vi "SetParam.vi"(6 "DAQmx Device Name":tag, 7 "RS":bool, 8 "error in (no error)":errorcluster, 9 "Param to Set in":u16, 10 "Visa":refnum<visa-resource-name>, 11 "Filein":string) -> (0 "error out":errorcluster)   [LabVIEW 2017]
uses:
  <vilib>/Utility/miscctls.llb/LVMinMaxIncTypeDef.ctl
  <vilib>/Utility/config.llb/NI_LVConfig.lvlib
  <vilib>/Utility/config.llb/Read Key (String).vi
panel:
  out "match substring":string
  out "RS Out":string
  out "Horizontal Progress Bar":i32(slide) min=0 max=32 scale=0.0..50.0
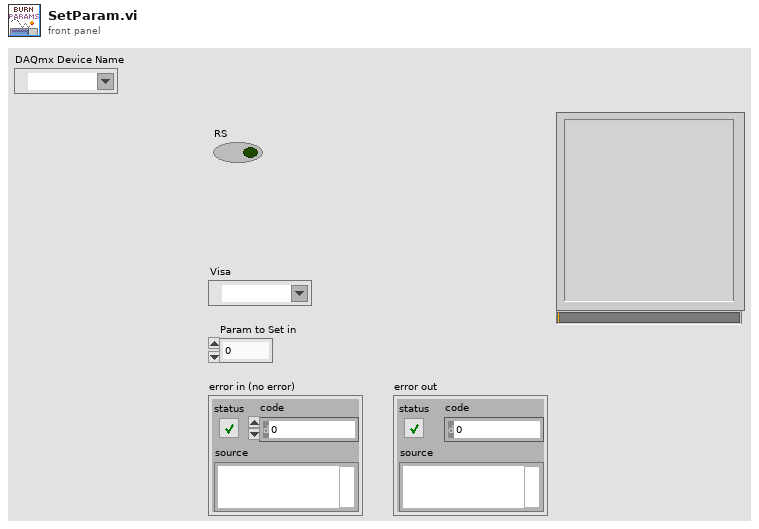
[diagram p1: front panel]
types:
  T1 = typedef "NI_LVConfig.lvlib/Config Data RefNum.ctl" = refnum<k1>
  T2 = typedef "LVMinMaxIncTypeDef.ctl" = cluster{"Minimum":dbl, "Maximum":dbl, "Increment":dbl}
  T3 = cluster{"Action":string, "ON(T)OFF(F)":bool, "Func":enum16{"Init", "VEnable", "PowerOnOff", "PowerONVEnable"}}
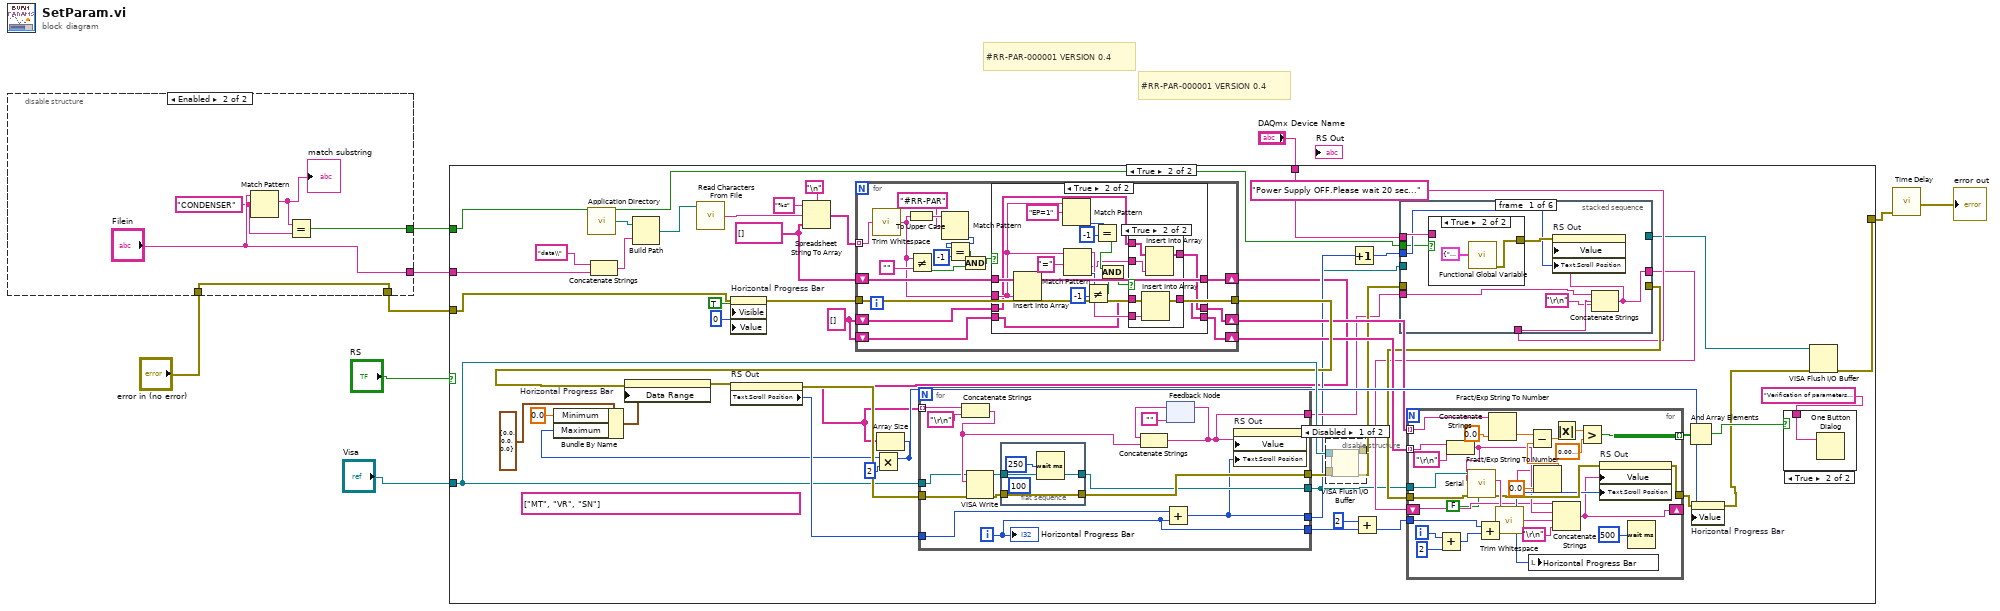
[diagram p0: block diagram]
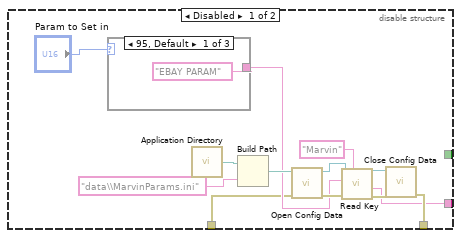
[diagram p2: hidden frame]
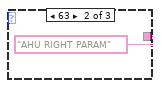
[diagram p3: hidden frame]
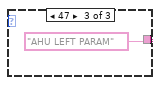
[diagram p4: hidden frame]
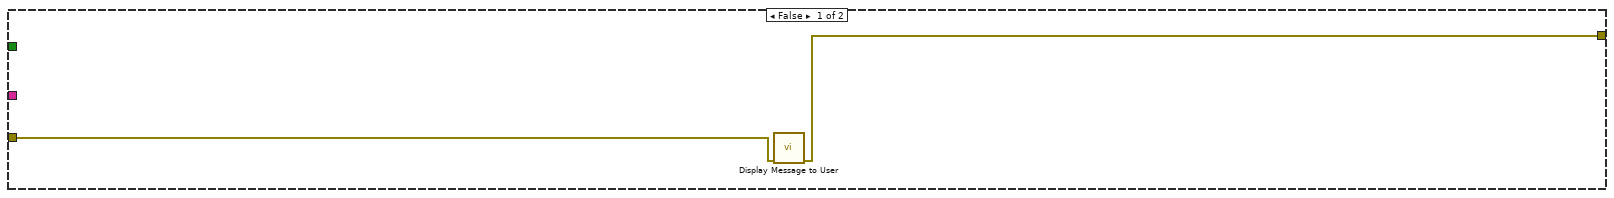
[diagram p5: hidden frame]
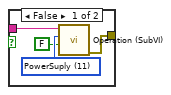
[diagram p7: hidden frame]
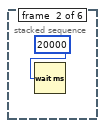
[diagram p8: hidden frame]
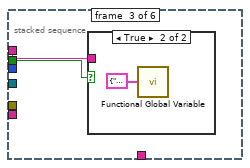
[diagram p9: hidden frame]
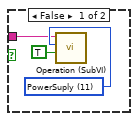
[diagram p10: hidden frame]
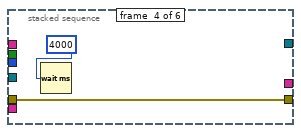
[diagram p11: hidden frame]
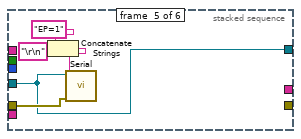
[diagram p12: hidden frame]
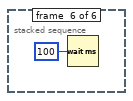
[diagram p13: hidden frame]
diagram:
  # "#RR-PAR-000001 VERSION 0.4"
  # "#RR-PAR-000001 VERSION 0.4"
  n1 = disable-structure shown="Enabled" {
    disable-tunnel: "error in (no error)" -> [w13 w30]
    disable-tunnel: [w12 w30] -> w6
    disable-tunnel: [w11 "Filein"] -> w5
    disable-tunnel: [_ w26] -> w1
    frame Disabled {
      n2 = case shown="95, Default" "Param to Set in" {
        tunnel: ["EBAY PARAM" ("section") "AHU RIGHT PARAM" ("section") "AHU LEFT PARAM" ("section")] -> w14
        frame 95, Default {
        }
        frame 63 {
        }
        frame 47 {
        }
      }
      n3 = call <vilib>:"Application Directory.vi"() -> ("Application Directory"=w22:path)
      n4 = Build Path(base path=w22, name or relative path="data\\MarvinParams.ini") -> (appended path=w18:path)
      n5 = call <vilib>:"Open Config Data.vi"("error in (no error)"=w13, "configuration file path"=w18) -> ("error out"=w17:errorcluster, "refnum"=w20:T1)  [unwired: 1 in, 7 out]
      n6 = call-poly <vilib>:"Read Key.vi"("section"="Marvin", "error in (no error)"=w17, "key"=w14, "refnum"=w20) -> ("error out"=w16:errorcluster, "value"=w11:string, "refnum out"=w15:T1)  [unwired: 2 in, 3 out]
      n7 = call <vilib>:"Close Config Data.vi"("error in (no error)"=w16, "refnum"=w15) -> ("error out"=w12:errorcluster)  [unwired: 8 in, 1 out]
    }
    frame Enabled {
      w27 = "CONDENSER" ("regular expression")
      n8 = Match Pattern(string="Filein", regular expression=w27) -> (match substring=w28:string)  [unwired: 1 in, 3 out]
      "match substring" <- w28
      n9 = Equal?(x=w28, y=w27) -> (x = y?=w26:bool)
    }
  }
  n10 = case shown="True" "RS" {
    tunnel: w6 -> [w32 w72]
    tunnel: [w31 w35] -> w9
    tunnel: "Visa" -> [_ w73]
    tunnel: w5 -> [_ w39]
    tunnel: "DAQmx Device Name" -> [_ w53]
    tunnel: w1 -> [_ w33]
    frame False {
      n11 = call "Display Message to User"("error in (no error)"=w32) -> ("error out"=w31:errorcluster)  [unwired: 9 in, 1 out]
    }
    frame True {
      w59 = string[] []
      w60 = string[] []
      (unwired) string[] ["MT", "VR", "SN"] ("array")
      n12 = call <vilib>:"Application Directory.vi"() -> ("Application Directory"=w70:path)
      n13 = Concatenate Strings("data\\" ("name or relative path"), w39) -> (w71:string)
      n14 = Build Path(base path=w70, name or relative path=w71) -> (appended path=w68:path)
      n15 = call <vilib>:"Read Characters From File.vi"("file path (dialog if empty)"=w68) -> ("character string"=w66:string)  [unwired: 5 in, 3 out]
      n16 = property on="Horizontal Progress Bar" class="Slide (strict)"(error in=w72, "Visible"=TRUE, "Value"=u8 0 ("Horizontal Progress Bar")) -> (error out=w64:errorcluster)  [unwired: 1 in, 1 out]
      n17 = Spreadsheet String To Array(delimiter (Tab)="\n", format string="%s", spreadsheet string=w66, array type (2D Dbl)=w60) -> (array=w65:string[])
      n18 = for {
        tunnel: w65 -> [w159] mode=indexing
        tunnel: w64 -> [w160]
        tunnel: [w160] -> w63
        shift-right: [w157] -> w37
        shift-left: w60 -> [w158]
        shift-right: [w146] -> w58
        shift-left: w59 -> [w147]
        shift-right: [w144] -> w57
        shift-left: w59 -> [w145]
        n19 = call <vilib>:"Trim Whitespace.vi"("string"=w159) -> ("trimmed string"=w148:string)  [unwired: 1 in]
        n20 = To Upper Case(1:w148) -> (0:w156:string)
        n21 = Not Equal?(x=w148, y="") -> (x != y?=w149:bool)
        n22 = Match Pattern(string=w156, regular expression="#RR-PAR") -> (offset past match=w154:i32)  [unwired: 1 in, 3 out]
        n23 = Equal?(x=w154, y=-1) -> (x = y?=w152:bool)
        n24 = And(x=w152, y=w149) -> (x .and. y?=w151:bool)
        n25 = case shown="True" w151 {
          tunnel: w158 -> [w163 w181]
          tunnel: [w163 w180] -> w157
          tunnel: w148 -> [_ w168]
          tunnel: w147 -> [w162 w164]
          tunnel: [w162 w165] -> w146
          tunnel: w145 -> [w161 w167]
          tunnel: [w161 w166] -> w144
          frame False {
          }
          frame True {
            n26 = Insert Into Array(array=w181, new element=w168) -> (w180:string[])  [unwired: 1 in]
            n27 = Match Pattern(string=w168, regular expression="EP=1") -> (offset past match=w177:i32)  [unwired: 1 in, 3 out]
            n28 = Match Pattern(string=w168, regular expression="=") -> (before substring=w178:string, after substring=w173:string, offset past match=w179:i32)  [unwired: 1 in, 1 out]
            n29 = Not Equal?(x=w179, y=-1) -> (x != y?=w176:bool)
            n30 = Equal?(x=w177, y=-1) -> (x = y?=w174:bool)
            n31 = And(x=w174, y=w176) -> (x .and. y?=w175:bool)
            n32 = case shown="True" w175 {
              tunnel: w167 -> [w183 w189]
              tunnel: [w183 w188] -> w166
              tunnel: w178 -> [_ w187]
              tunnel: w173 -> [_ w186]
              tunnel: w164 -> [w182 w185]
              tunnel: [w182 w184] -> w165
              frame False {
              }
              frame True {
                n33 = Insert Into Array(array=w189, new element=w187) -> (w188:string[])  [unwired: 1 in]
                n34 = Insert Into Array(array=w185, new element=w186) -> (w184:string[])  [unwired: 1 in]
              }
            }
          }
        }
      }
      n35 = Array Size(array=w37) -> (size(s)=w67:i32)
      n36 = Multiply(x=w67, y=2) -> (x*y=w50:i32)
      n37 = Bundle By Name(cluster=T2 {"Minimum"=0.0, "Maximum"=0.0, "Increment"=0.0} ("Data Entry Limits"), "Minimum"=0.0, "Maximum"=w50) -> (w79:T2)
      n38 = property on="Horizontal Progress Bar" class="Slide (strict)"(error in=w63, "Data Range"=w79) -> (error out=w76:errorcluster)  [unwired: 1 in, 1 out]
      n39 = property on="RS Out" class="Str"(error in=w76) -> (error out=w75:errorcluster, "Text.Scroll Position"=w74:u32)  [unwired: 1 in, 1 out]
      n40 = for {
        tunnel: w37 -> [w200] mode=indexing
        tunnel: w75 -> [w204]
        tunnel: [w197] -> w77
        tunnel: w74 -> [w196]
        tunnel: w73 -> [w195]
        tunnel: [w193] -> w38
        tunnel: [w192] -> w47
        tunnel: [w191] -> w45
        tunnel: [w190] -> w43
        i -> [w192]
        n41 = Concatenate Strings(w200, "\r\n" ("string")) -> (w198:string)
        n42 = VISA Write(VISA resource name=w195, write buffer=w198, error in (no error)=w204) -> (VISA resource name out=w194:refnum<visa-resource-name>, error out=w203:errorcluster)  [unwired: 1 out]
        n43 = flat-sequence {
          tunnel: w203 -> [w206]
          tunnel: [w206] -> w197
          tunnel: w194 -> [w205]
          tunnel: [w205] -> w193
          frame #0 {
            (unwired) u32 100 ("milliseconds to wait")
            n44 = Wait (ms)(milliseconds to wait=u32 250) -> ()  [unwired: 1 out]
          }
        }
        n45 = Add(x=w196, y=w192) -> (x+y=w190:u32)
        n46 = feedback #1("") -> (w202:string)
        n47 = Concatenate Strings(w202, w198) -> (w191:string)
        n48 = feedback-in #1(w191) -> ()
        n49 = property on="RS Out" class="Str"("Value"=w191, "Text.Scroll Position"=w190) -> ()  [unwired: 2 in, 2 out]
        "Horizontal Progress Bar" <- w192
      }
      n50 = disable-structure shown="Disabled" {
        disable-tunnel: w77 -> [w85 _]
        disable-tunnel: w73 -> [w84 _]
        disable-tunnel: [w83 _] -> w52
        frame Disabled {
          n51 = VISA Flush I/O Buffer(VISA resource name=w84, error in (no error)=w85) -> (error out=w83:errorcluster)  [unwired: 1 in, 1 out]
        }
        frame Enabled {
        }
      }
      n52 = Increment(x=w43) -> (x+1=w42:u32)
      n53 = Add(x=2, y=w47) -> (x+y=w41:i32)
      n54 = stacked-sequence {
        tunnel: w53 -> [w93 _ w102 _ _ _]
        tunnel: [_ _ _ w107 _ _] -> w51
        tunnel: w52 -> [_ _ _ w107 w113 _]
        tunnel: "Power Supply OFF.Please wait 20 sec..." ("message") -> [w91 _ _ _ _ _]
        tunnel: w45 -> [w89 _ _ _ _ _]
        tunnel: [w88 _ _ _ _ _] -> w44
        tunnel: w42 -> [w87 _ _ _ _ _]
        tunnel: w38 -> [_ _ _ _ w109 _]
        tunnel: [_ _ _ _ w109 _] -> w34
        tunnel: w33 -> [w86 _ w101 _ _ _]
        frame #0 {
          n55 = case shown="True" w86 {
            tunnel: w93 -> [w95 _]
            tunnel: [w94 w98] -> w92
            frame False {
              w97 = u16 11 items=["Init", "0 ohm", "6 ohm", "13.2 ohm", "15 ohm", "25.9 ohm", "33 ohm", "Down", "Up", "Venable", "Firmware", "PowerSuply"] ("Operation")
              n56 = call "Operation (SubVI).vi"("On/Off"=FALSE, "Operation"=w97, "DAQmx Device Name"=w95) -> ("error out"=w94:errorcluster)  [unwired: 8 in]
            }
            frame True {
              n57 = call "Functional Global Variable.vi"("Operation"=T3 {"Action"="Modify", "ON(T)OFF(F)"=FALSE, "Func"=enum."PowerOnOff"}) -> ("error out"=w98:errorcluster)  [unwired: 8 in, 2 out]
            }
          }
          n58 = Concatenate Strings(w89, w91, "\r\n") -> (w88:string)
          n59 = property on="RS Out" class="Str"(error in=w92, "Value"=w88, "Text.Scroll Position"=w87) -> ()  [unwired: 1 in, 2 out]
        }
        frame #1 {
          n60 = Wait (ms)(milliseconds to wait=u32 20000) -> ()  [unwired: 1 out]
        }
        frame #2 {
          n61 = case shown="True" w101 {
            tunnel: w102 -> [w103 _]
            frame False {
              w104 = u16 11 items=["Init", "0 ohm", "6 ohm", "13.2 ohm", "15 ohm", "25.9 ohm", "33 ohm", "Down", "Up", "Venable", "Firmware", "PowerSuply"] ("Operation")
              n62 = call "Operation (SubVI).vi"("On/Off"=TRUE, "Operation"=w104, "DAQmx Device Name"=w103) -> ()  [unwired: 8 in, 1 out]
            }
            frame True {
              n63 = call "Functional Global Variable.vi"("Operation"=T3 {"Action"="Modify", "ON(T)OFF(F)"=TRUE, "Func"=enum."PowerOnOff"}) -> ()  [unwired: 8 in, 3 out]
            }
          }
        }
        frame #3 {
          n64 = Wait (ms)(milliseconds to wait=u32 4000) -> ()  [unwired: 1 out]
        }
        frame #4 {
          n65 = Concatenate Strings("EP=1", "\r\n" ("string")) -> (w110:string)
          n66 = call "Serial.vi"("error in (no error)"=w113, "write buffer"=w110, "VISA resource name"=w109) -> ()  [unwired: 7 in, 2 out]
        }
        frame #5 {
          n67 = Wait (ms)(milliseconds to wait=u32 100) -> ()  [unwired: 1 out]
        }
      }
      n68 = for {
        tunnel: w38 -> [w143]
        tunnel: w57 -> [w141] mode=indexing
        tunnel: w51 -> [w140]
        tunnel: w58 -> [w138] mode=indexing
        tunnel: [w127] -> w48
        tunnel: [w130] -> w56 mode=indexing
        tunnel: w41 -> [w129]
        shift-right: [w123] -> _
        shift-left: w44 -> [w124]
        i -> [w121]
        n69 = Add(x=w121, y=2) -> (x+y=w119:i32)
        n70 = Concatenate Strings(w141, "\r\n" ("string")) -> (w125:string)
        n71 = call "Serial.vi"("Close"=FALSE, "error in (no error)"=w140, "write buffer"=w125, "VISA resource name"=w143) -> ("error out"=w128:errorcluster, "read buffer"=w139:string)  [unwired: 6 in]
        n72 = Add(x=w129, y=w119) -> (x+y=w126:i32)
        n73 = Fract/Exp String To Number(string=w138, default (0 dbl)=sgl 0.0 ("default (0 DBL)")) -> (number=w135:sgl)  [unwired: 2 in, 1 out]
        n74 = call <vilib>:"Trim Whitespace.vi"("string"=w139) -> ("trimmed string"=w117:string)  [unwired: 1 in]
        n75 = local write "Horizontal Progress Bar"(w126) -> ()
        n76 = Fract/Exp String To Number(string=w117, default (0 dbl)=sgl 0.0 ("default (0 DBL)")) -> (number=w134:sgl)  [unwired: 2 in, 1 out]
        n77 = Subtract(x=w135, y=w134) -> (x-y=w133:sgl)
        n78 = Absolute Value(x=w133) -> (abs(x)=w132:sgl)
        n79 = Concatenate Strings(w124, w125, w117, "\r\n") -> (w123:string)
        n80 = Greater?(x=w132, y=sgl 0.01) -> (0:w130:bool)
        n81 = property on="RS Out" class="Str"(error in=w128, "Value"=w123, "Text.Scroll Position"=w126) -> (error out=w127:errorcluster)  [unwired: 1 in, 1 out]
        n82 = Wait (ms)(milliseconds to wait=u32 500) -> ()  [unwired: 1 out]
      }
      n83 = And Array Elements(Boolean array=w56) -> (logical AND=w55:bool)
      n84 = property on="Horizontal Progress Bar" class="Slide (strict)"(error in=w48, "Value"=w67) -> (error out=w36:errorcluster)  [unwired: 1 in, 1 out]
      n85 = case shown="True" w55 {
        tunnel: "Verification of parameters failed !" ("message") -> [_ w115]
        frame False {
        }
        frame True {
          n86 = One Button Dialog(message=w115) -> ()  [unwired: 1 in, 1 out]
        }
      }
      n87 = VISA Flush I/O Buffer(VISA resource name=w34, error in (no error)=w36) -> (error out=w35:errorcluster)  [unwired: 1 in, 1 out]
    }
  }
  n88 = call "Time Delay"("error in (no error)"=w9) -> ("error out"=→"error out":errorcluster)  [unwired: 10 in]
